vi "WebSocket Do Handshake.vi"(8 "error in (no error)":errorcluster, 9 "timeout ms (5000)":i32=5000, 11 "WebSocket Connection in":refnum<k5>) -> (0 "error out":errorcluster, 1 "Request URI":string, 2 "Headers Out":variant, 3 "WebSocket Connection out":refnum<k5>)   [LabVIEW 2018]
doc: "Performs the WebSockets HTTP handshaking on the new TCP connection. The client sends HTTP headers and the server must reply with a correctly formed HTTP response.\nWebSockets API 1.3.0.13\nSam Sharp - Intelligent Energy\nCopyright (c) 2015, Intelligent Energy"
panel:
  out "HTTP Headers":string
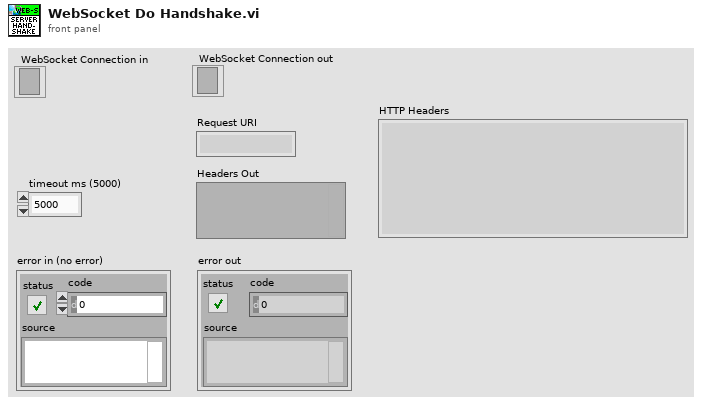
[diagram p1: front panel]
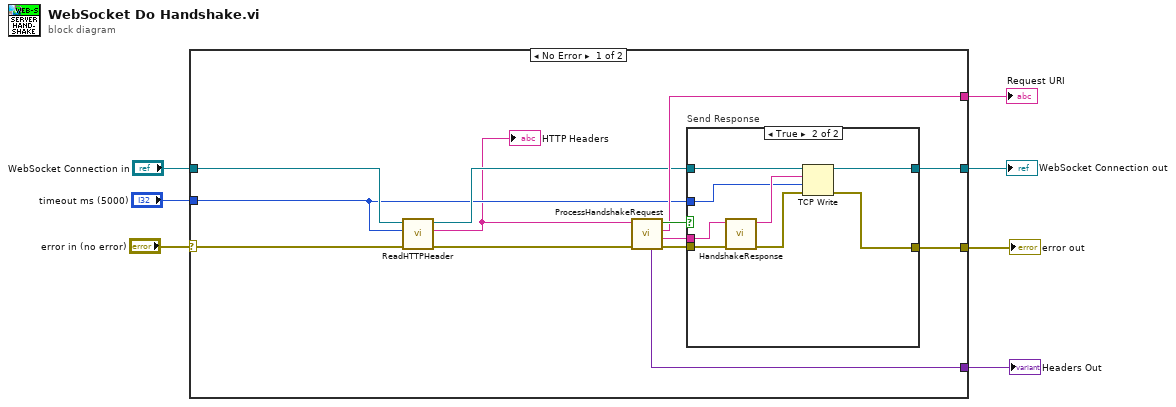
[diagram p0: block diagram]
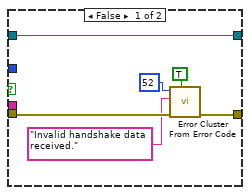
[diagram p2: hidden frame]
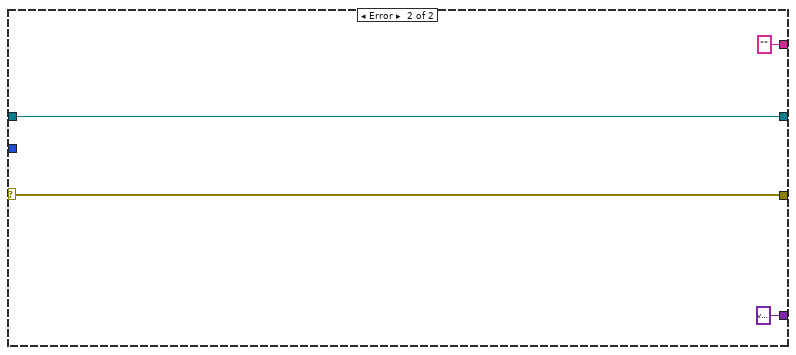
[diagram p3: hidden frame]
diagram:
  n1 = case shown="No Error" "error in (no error)" {
    selector: "error in (no error)" -> [w12 w38]
    tunnel: [w20 w37] -> w7
    tunnel: "WebSocket Connection in" -> [w13 w37]
    tunnel: [w16 w38] -> w4
    tunnel: "timeout ms (5000)" -> [w9 _]
    tunnel: [w15 variant ("Headers Out")] -> w2
    tunnel: [w14 "" ("Path")] -> w1
    frame No Error {
      n2 = call "ReadHTTPHeader.vi"("error in (no error)"=w12, "timeout ms (25000)"=w9, "WebSocket Connection in"=w13) -> ("error out"=w11:errorcluster, "HTTP Header"=w8:string, "WebSocket Connection out"=w10:refnum<k5>)  [unwired: 6 in]
      "HTTP Headers" <- w8
      n3 = call "ProcessHandshakeRequest.vi"("error in (no error)"=w11, "HTTP Headers"=w8) -> ("error out"=w17:errorcluster, "Sec-WebSocket-Key"=w19:string, "Path"=w14:string, "Is Websocket Request?"=w18:bool, "Headers Out"=w15:variant)  [unwired: 4 in, 1 out]
      n4 = case "Send Response" shown="True" w18 {
        tunnel: w19 -> [_ w34]
        tunnel: w10 -> [w26 w32]
        tunnel: [w26 w31] -> w20
        tunnel: w17 -> [w24 w29]
        tunnel: [w25 w28] -> w16
        tunnel: w9 -> [_ w27]
        frame False {
          n5 = call <vilib>:"Error Cluster From Error Code.vi"("show call chain? (False)"=TRUE, "error in (no error)"=w24, "error message (\"\")"="Invalid handshake data received." ("error message (\"\")"), "error code (0)"=52) -> ("error out"=w25:errorcluster)  [unwired: 5 in]
        }
        frame True {
          n6 = call "HandshakeResponse.vi"("error in (no error)"=w29, "Sec-WebSocket-Key"=w34) -> ("error out"=w30:errorcluster, "Response Headers"=w33:string)  [unwired: 8 in]
          n7 = TCP Write(connection ID=w32, data in=w33, error in (no error)=w30, 9:w27) -> (connection ID out=w31:refnum<k5>, error out=w28:errorcluster)  [unwired: 1 out]
        }
      }
    }
    frame Error {
    }
  }
  "WebSocket Connection out" <- w7
  "error out" <- w4
  "Headers Out" <- w2
  "Request URI" <- w1
